vi "Ejercicio_20_Banda_Transportadora.vi"() -> ()   [LabVIEW 2020]
panel:
  in  "stop":bool
  in  "Knob":dbl(knob) scale=0.0..10.0
  out "Slide":dbl(slide) scale=0.0..10.0
  out "Boolean 2":bool
  in  "Boolean":bool
  # "Aqui lo unico que se cambia es la presentacion de los componentes \na usar, esto con las imagenes previemente descargadas del complemento"
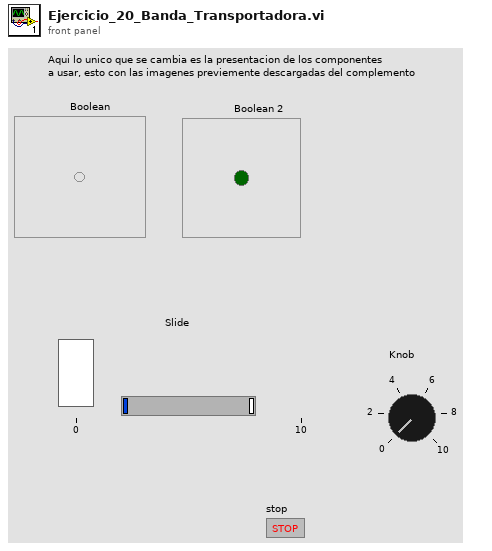
[diagram p1: front panel]
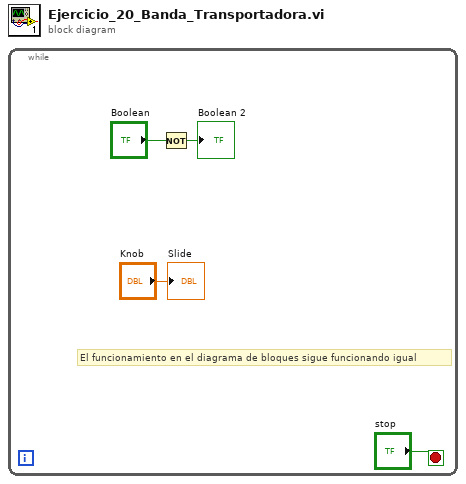
[diagram p0: block diagram]
diagram:
  n1 = while {
    stop <- "stop" stop-if-true
    # "El funcionamiento en el diagrama de bloques sigue funcionando igual"
    n2 = Not(x="Boolean") -> (.not. x?=→"Boolean 2":bool)
    "Slide" <- "Knob"
  }
